vi "Sort_Alarm_Status.vi"(11 "Array in":bool[](array[boolean])) -> (3 "Array out":bool[](array[boolean]))   [LabVIEW 2018]
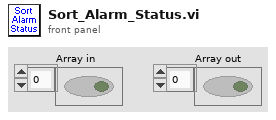
[diagram p1: front panel]
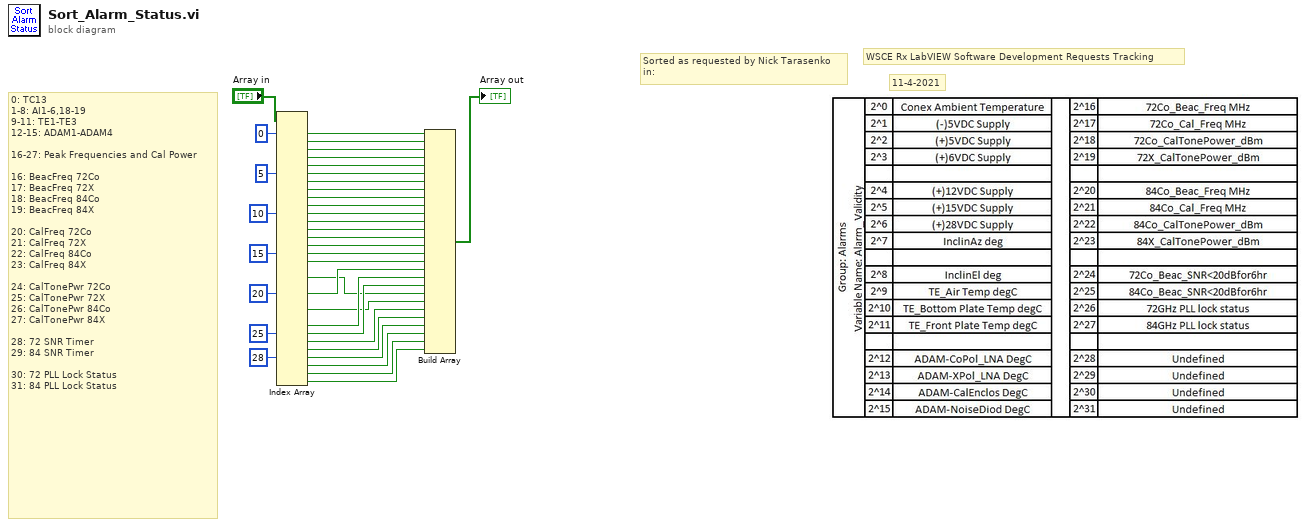
[diagram p0: block diagram]
diagram:
  # "11-4-2021"
  # "WSCE Rx LabVIEW Software Development Requests Tracking"
  # "Sorted as requested by Nick Tarasenko\nin:"
  # "0: TC13\n1-8: AI1-6,18-19\n9-11: TE1-TE3\n12-15: ADAM1-ADAM4\n\n16-27: Peak Frequencies and Cal Power\n\n16: BeacFreq 72Co \n17: BeacFreq 72X \n18: BeacFreq 84Co \n19: BeacFreq 84X\n \n20: CalFreq 72Co\n21: CalFreq 72X\n22: CalFreq 84Co\n23: CalFreq 84X\n \n24: CalTonePwr 72Co\n25: CalTonePwr 72X\n26: CalTonePwr 84Co\n27: CalTonePwr 84X\n\n28: 72 SNR Timer\n29: 84 SNR Timer\n\n30: 72 PLL Lock Status\n31: 84 PLL Lock Status"
  n1 = Index Array(array="Array in", index #1=0 ("index"), index #6=5 ("index"), index #11=10 ("index"), index #16=15 ("index"), index #21=20 ("index"), index #26=25 ("index"), index #29=28 ("index")) -> (element #1=w37:bool, element #2=w27:bool, element #3=w26:bool, element #4=w25:bool, element #5=w24:bool, element #6=w23:bool, element #7=w22:bool, element #8=w21:bool, element #9=w20:bool, element #10=w19:bool, element #11=w18:bool, element #12=w17:bool, element #13=w16:bool, element #14=w15:bool, element #15=w14:bool, element #16=w13:bool, element #17=w1:bool, element #19=w9:bool, element #21=w12:bool, element #23=w8:bool, element #25=w11:bool, element #26=w10:bool, element #27=w7:bool, element #28=w6:bool, element #29=w5:bool, element #30=w4:bool, element #31=w3:bool, element #32=w2:bool)  [unwired: 25 in, 4 out]
  n2 = Build Array(w37, w27, w26, w25, w24, w23, w22, w21, w20, w19, w18, w17, w16, w15, w14, w13, w1, w12, w11, w10, w9, w8, w7, w6, w5, w4, w3, w2) -> (→"Array out":bool[])
